vi "QMH - Polymorphic.vi"   [LabVIEW 2024, in "QMH Messaging.lvlib"]
uses:
  QMH Messaging.lvlib
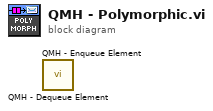
[diagram p0: block diagram]
diagram:
  n1 = call "QMH - Dequeue Element.vi"() -> ()  [unwired: 8 in, 4 out]
  n2 = call "QMH - Enqueue Element.vi"() -> ()  [unwired: 10 in, 2 out]
